vi "Post-Actor.vi"(8 "error in (no error)":errorcluster, 11 "Instruments in":refnum<class "Instruments.lvclass">) -> (0 "error out":errorcluster, 3 "Instruments out":refnum<class "Instruments.lvclass">)   [LabVIEW 2023, in "Instruments.lvlib" / "Instruments.lvclass"]
doc: "<b>Post Actor Init </b>\nThis routine is called in the Post Launch Initialize routine.\n\nIt is provided as a means to provide the necessary hooks to perform actions <b> after</b> the the remainder of the actor has been initialized. A common use case is to schedule periodic messages (such as polling)\n\n<b> Instrument </b>\nThis routine schedules the polling message"
uses:
  Library/Instruments.lvclass
  Library/Instruments.lvclass/Instruments.ctl
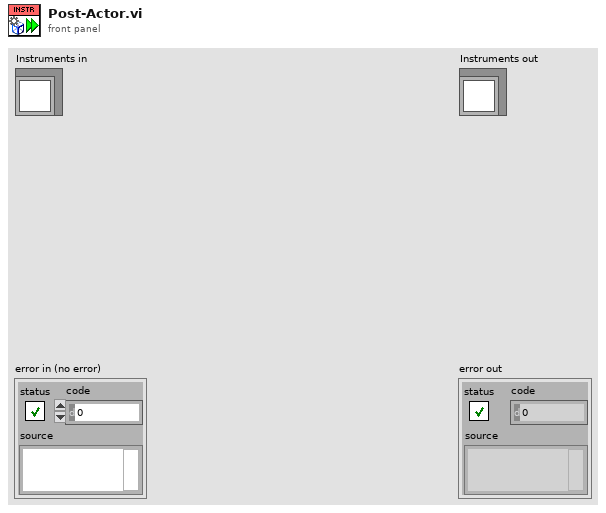
[diagram p1: front panel]
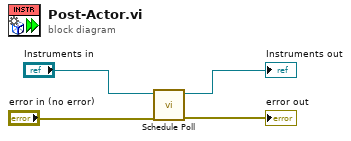
[diagram p0: block diagram]
diagram:
  n1 = call "Schedule Poll.vi"("error in (no error)"="error in (no error)", "Instruments in"="Instruments in") -> ("error out"=→"error out":errorcluster, "Instruments out"=→"Instruments out":refnum<class "Instruments.lvclass">)  [unwired: 8 in]
